vi "FlatToRichcif_template_Statistics.vi"(5 "OutputClusterType":T1, 11 "InputCluster":T2) -> (3 "OutputCluster":T1)   [LabVIEW 2021, in "Template_client.lvlib"]
uses:
  Template_client.lvlib
  cif_template_Statistics_Flat.ctl
  cif_template_Statistics.ctl
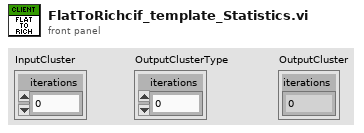
[diagram p1: front panel]
types:
  T1 = typedef "Template_client.lvlib/cif_template_Statistics.ctl" = cluster{"iterations":u64}
  T2 = typedef "Template_client.lvlib/cif_template_Statistics_Flat.ctl" = cluster{"iterations":u64}
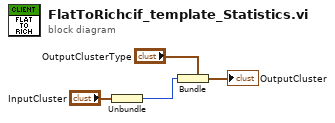
[diagram p0: block diagram]
diagram:
  n1 = Unbundle "Unbundle"("InputCluster") -> ("iterations"=w1:u64)
  n2 = Bundle "Bundle"(cluster="OutputClusterType", "iterations"=w1) -> (→"OutputCluster":T1)
